vi "Return Error Report.vi"(8 "error in (no error)":errorcluster, 10 "error Source(No Error)":errorcluster, 11 "Console Error(Console2API) in":refnum<class "Console Reply Error Report.lvclass">) -> (0 "error out":errorcluster, 3 "Console Error(Console2API) out":refnum<class "Console Reply Error Report.lvclass">)   [LabVIEW 2015, in "EditPanel API.lvlib" / "Console Reply Error Report.lvclass"]
uses:
  Console Reply Error Report.lvclass
  Console Reply Error Report.lvclass/Console Reply Error Report.ctl
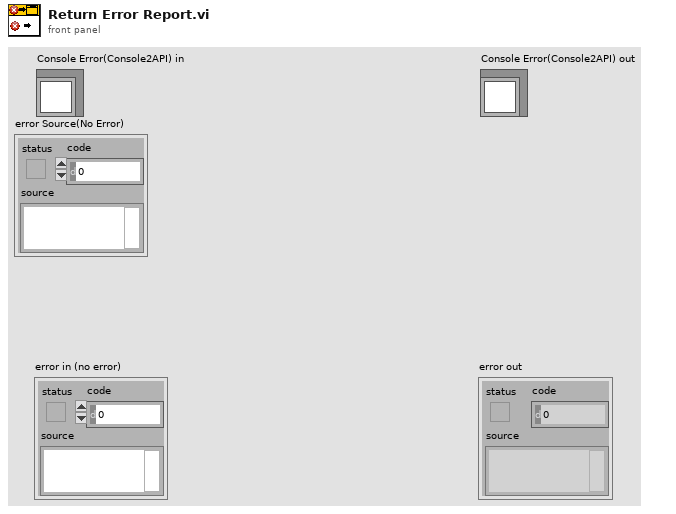
[diagram p1: front panel]
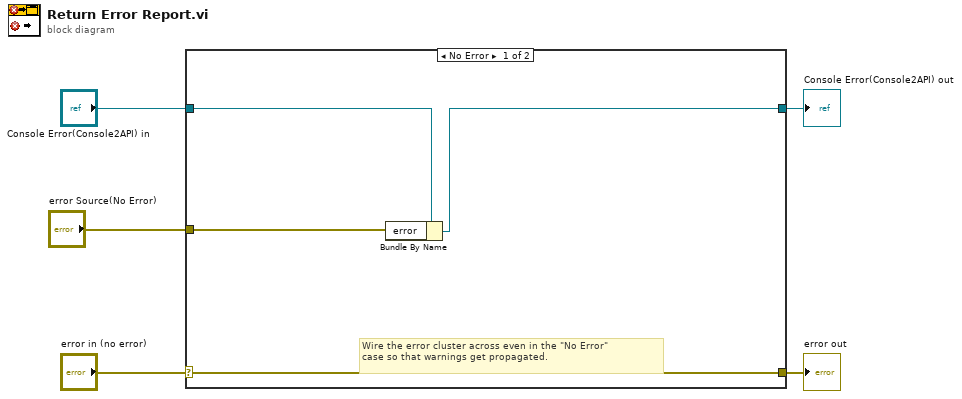
[diagram p0: block diagram]
diagram:
  n1 = case shown="No Error" "error in (no error)" {
    selector: "error in (no error)" -> [w9 w11]
    tunnel: [w9 w11] -> w4
    tunnel: [w6 w10] -> w2
    tunnel: "Console Error(Console2API) in" -> [w8 w10]
    tunnel: "error Source(No Error)" -> [w7 _]
    frame No Error {
      # "Wire the error cluster across even in the \"No Error\"\ncase so that warnings get propagated."
      n2 = Bundle By Name(cluster=w8, "error"=w7) -> (w6:refnum<class "Console Reply Error Report.lvclass">)
    }
    frame Error {
    }
  }
  "error out" <- w4
  "Console Error(Console2API) out" <- w2
